vi "Construct PDU.vi"(6 "data":u8[](array[numeric]), 8 "error in":errorcluster, 9 "command":cluster{"type":string, "number":u8}={"type"="k", "number"=1}, 10 "source address":u8, 11 "target address":u8) -> (0 "error out":errorcluster, 3 "ELAN data unit out":refnum<class "ELAN PDU.lvclass">)   [LabVIEW 2021, in "ELAN PDU.lvclass"]
uses:
  ELAN PDU.lvclass
  ELAN PDU.lvclass/ELAN PDU.ctl
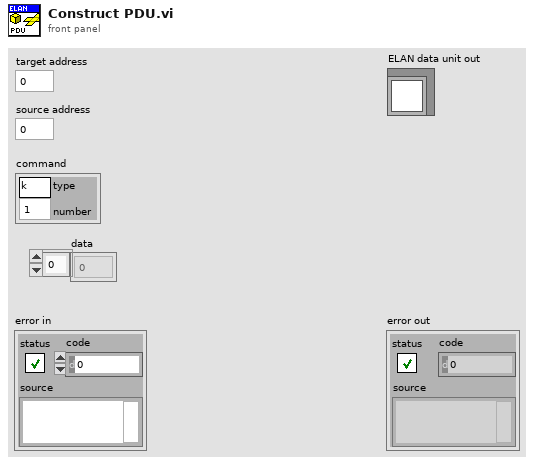
[diagram p1: front panel]
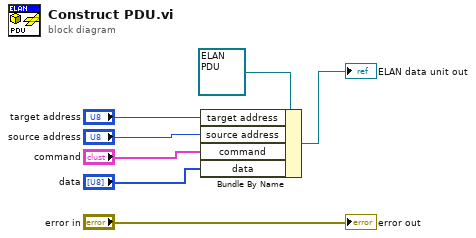
[diagram p0: block diagram]
diagram:
  n1 = Bundle By Name(cluster=refnum<class "ELAN PDU.lvclass"> refnum ("Modbus Data Unit"), "target address"="target address", "source address"="source address", "command"="command", "data"="data") -> (→"ELAN data unit out":refnum<class "ELAN PDU.lvclass">)
  "error out" <- "error in"
